vi "2022NewInstrumentationU6Revision.vi"() -> ()   [LabVIEW 2021]
uses:
  <vilib>/Analysis/baseanly.llb/Mean (DBL).vi
  <vilib>/Analysis/NI_AALBase.lvlib
panel:
  out "Combustion Chamber Pressure":dbl(knob) scale=0.0..10.0
  out "Pre-Injector Pressure":dbl(graph)
  out "Post-Combustion Chamber Temperature":dbl(knob) scale=0.0..10.0
  out "Pre-Combustion Chamber Temperature":dbl(knob) scale=0.0..100.0
  out "Injector Temperature":dbl(knob) scale=0.0..10.0
  out "Run Tank: Temperature":dbl(slide) scale=0.0..100.0
  out "Run Tank: Pressure":dbl(knob) scale=0.0..10.0
  out "N20 Post-Tank: Pressure":dbl(knob) scale=0.0..10.0
  out "N2 Post-tank: Pressure":dbl(knob) scale=0.0..10.0
  in  "file name":string
  in  "file path":path
  in  "Iterations/Second":i32=1
  in  "Binary":bool
  in  "StreamSettlingFactor":i32
  in  "Resolution Index":u8
  in  "Range Constants":u8[](array[ring])=[0, 0, 0, 0] items=["LJ_rgBIP10V", "LJ_rgBIP1V", "LJ_rgBIPP1V", "LJ_rgBIPP01V"]
  out "Stream Parameters":T1 {"Device Backlog [%]" format="%.2f"}
  in  "PC buffer size (seconds)":dbl=10.0 format="%.2f"
  in  "Scan List (-)":u8[](array[numeric])=[199, 199, 199, 199]
  in  "Scan List (+)":u8[](array[numeric])=[0, 1, 2, 3]
  out "# of iterations":i32
  in  "Scan Rate (Hz)":dbl=1000.0 format="%.3f"
  in  "stop":bool
  out "Error Message":string
  # "This example streams from the first found USB U6."
  # "The + scan list is the positive\nchannels.  For each element in\nthe + list, there must also be\nan element in the - list, which is\nthe negative channels.  For\nsingle-ended channels, put in\n199 for the negative channel.\n\nTo remove an element, right-click\non it, select Data Operations =>\nRemove Element.\n\nTo empty an array, right-click\nnear the edge, select Data\nOperations => Empty Array.\n\nOther useful operations:  From the\nOperate menu are \"Make Current\nValues Default\" and \"Reinitialize\nTo Default\"."
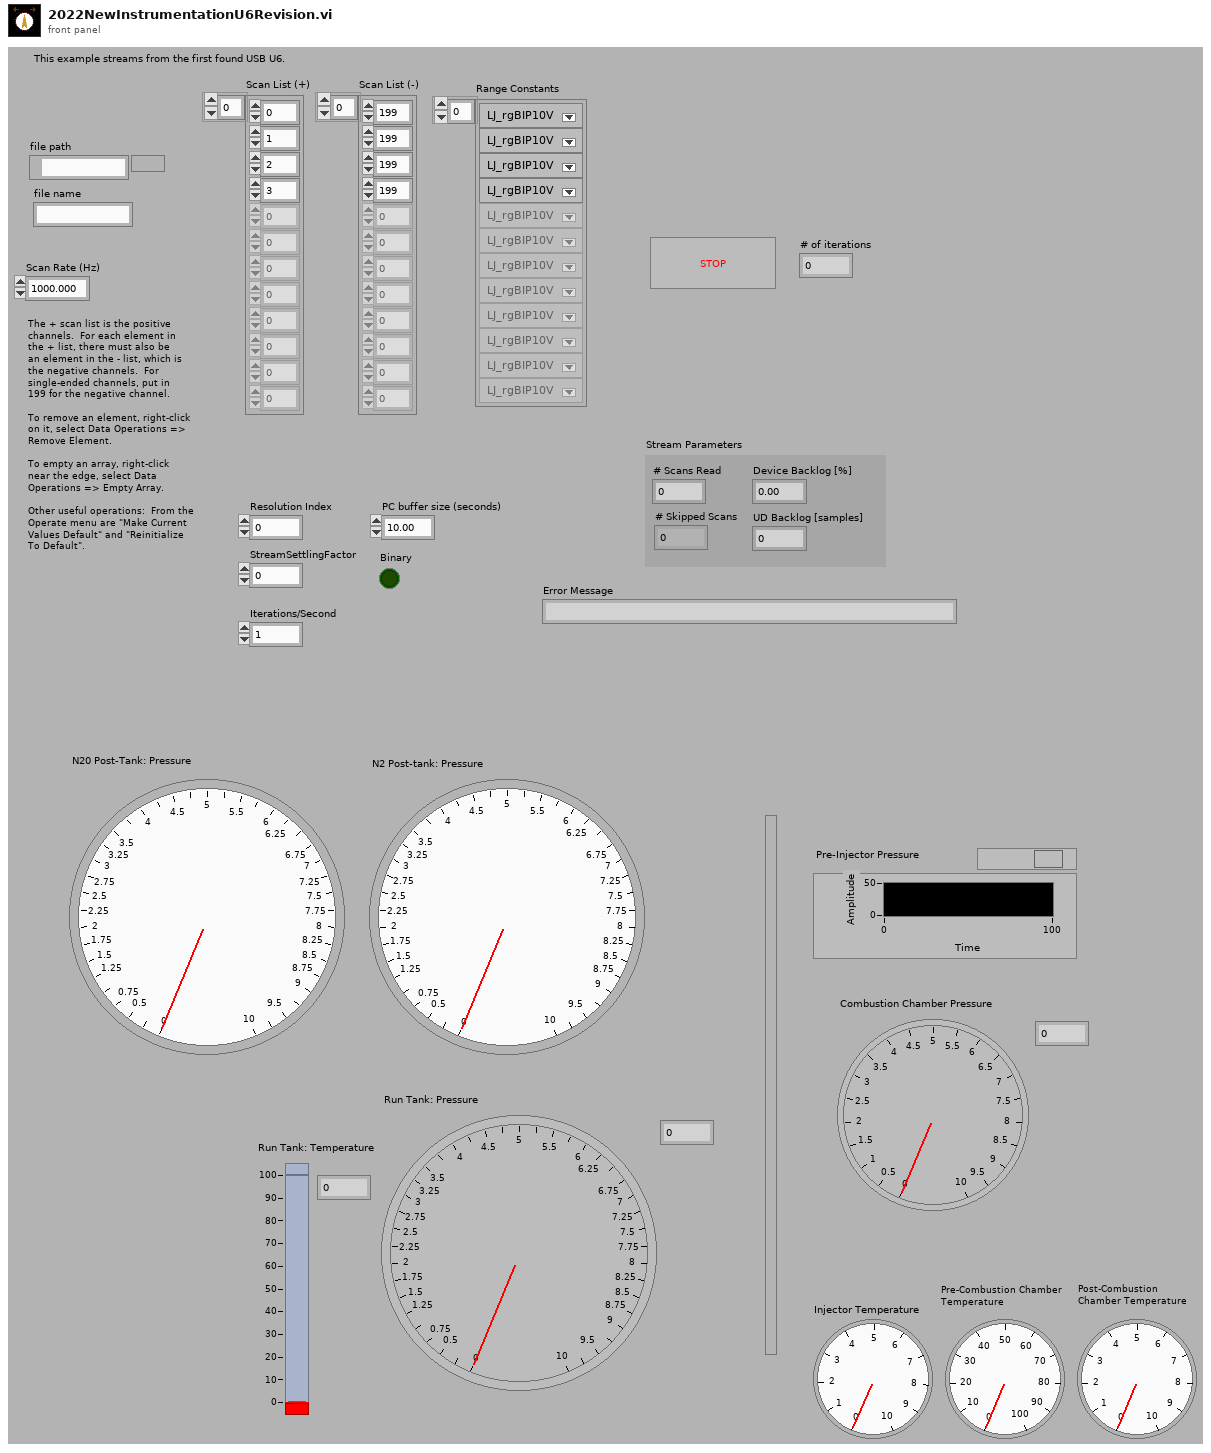
[diagram p1: front panel]
types:
  T1 = cluster{"# Scans Read":i32, "# Skipped Scans":i32, "Device Backlog [%]":dbl, "UD Backlog [samples]":i32}
  T2 = enum16{"open", "open or create", "create or replace", "create", "open (read-only)"}
  T3 = cluster{"PC buffer size (seconds)":dbl, "Resolution Index":u8, "StreamSettlingFactor":i32, "Binary":bool}
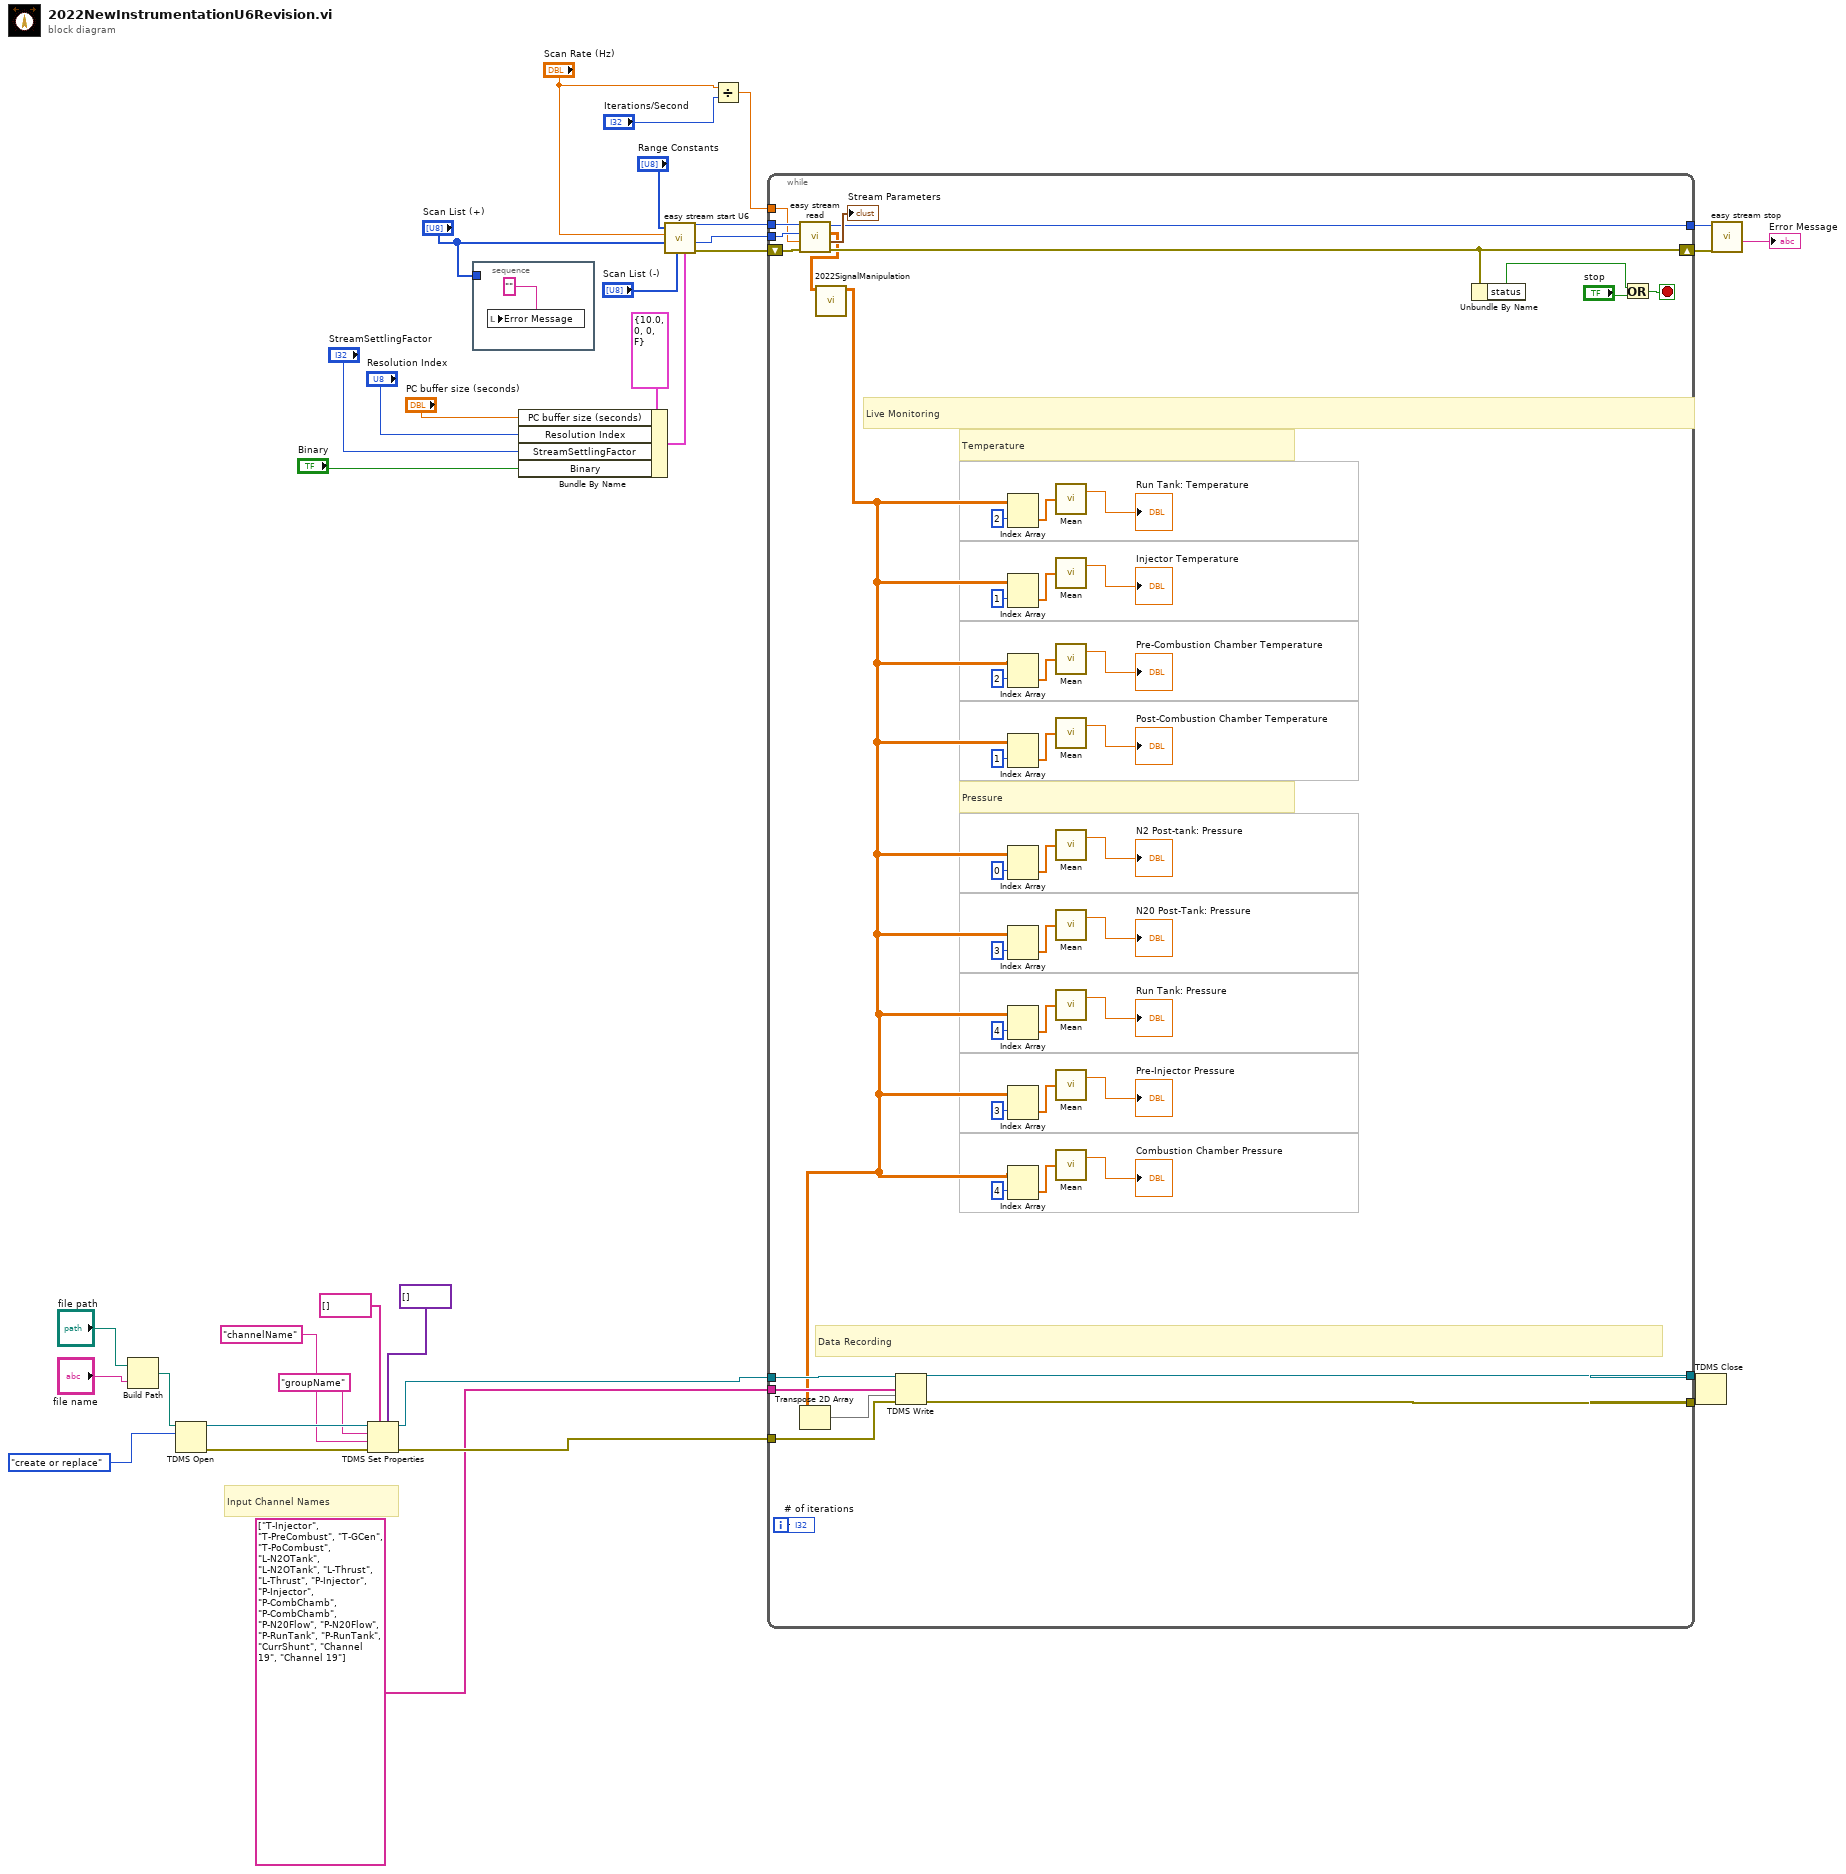
[diagram p0: block diagram]
diagram:
  # "Input Channel Names"
  n1 = Build Path(base path="file path", name or relative path="file name") -> (appended path=w11:path)
  n2 = TDMS Open(10:T2."create or replace" ("operation (0:open)"), 11:w11) -> (0:w16:errorcluster, 3:w15:refnum<k34>)  [unwired: 5 in]
  n3 = TDMS Set Properties(5:variant[] [] ("property values"), 7:string[] [] ("property names"), 8:w16, 9:"channelName" ("channel name"), 10:"groupName" ("group name"), 11:w15) -> (0:w6:errorcluster, 3:w5:refnum<k34>)  [unwired: 2 out]
  n4 = stacked-sequence {
    tunnel: "Scan List (+)" -> [_]
    frame #0 {
      n5 = local write "Error Message"("" ("Error Message")) -> ()
    }
  }
  n6 = Bundle By Name(cluster=T3 {"PC buffer size (seconds)"=10.0, "Resolution Index"=0, "StreamSettlingFactor"=0, "Binary"=FALSE} ("Advanced"), "PC buffer size (seconds)"="PC buffer size (seconds)", "Resolution Index"="Resolution Index", "StreamSettlingFactor"="StreamSettlingFactor", "Binary"="Binary") -> (w24:T3)
  n7 = call "easy stream start U6.vi"("Advanced"=w24, "Scan List (-)"="Scan List (-)", "Scan List (+)"="Scan List (+)", "Scan Rate (Hz)"="Scan Rate (Hz)", "Range Constants"="Range Constants") -> ("error out"=w33:errorcluster, "# Channels"=w32:i32, "Handle Out"=w31:i32)  [unwired: 3 in, 1 out]
  n8 = Divide(x="Scan Rate (Hz)", y="Iterations/Second") -> (x/y=w17:dbl)
  n9 = while {
    tunnel: w31 -> [w74]
    tunnel: w32 -> [w75]
    shift-left: w33 -> [w76]
    shift-right: [w56] -> w30
    tunnel: w17 -> [w72]
    tunnel: w6 -> [w71]
    tunnel: w5 -> [w70]
    tunnel: string[] ["T-Injector", "T-PreCombust", "T-GCen", "T-PoCombust", "L-N2OTank", "L-N2OTank", "L-Thrust", "L-Thrust", "P-Injector", "P-Injector", "P-CombChamb", "P-CombChamb", "P-N20Flow", "P-N20Flow", "P-RunTank", "P-RunTank", "CurrShunt", "Channel 19", "Channel 19"] -> [w69]
    tunnel: [w68] -> w3
    tunnel: [w67] -> w2
    tunnel: [w55] -> w1
    i -> [w77]
    stop <- w78 stop-if-true
    # "Data Recording"
    # "Temperature"
    # "Live Monitoring"
    # "Pressure"
    n10 = call "easy stream read.vi"("error in"=w76, "Scans To Read"=w72, "# Channels In Stream"=w75, "Handle In"=w74) -> ("error out"=w56:errorcluster, "Stream Parameters"=→"Stream Parameters":T1, "Data"=w54:dbl[][], "Handle Out"=w55:i32)  [unwired: 4 in]
    n11 = call "2022SignalManipulation.vi"("Data"=w54) -> ("Array"=w36:dbl[][])  [unwired: 10 in]
    n12 = Transpose 2D Array(2D array=w36) -> (transposed array=w66:dbl[][])
    n13 = TDMS Write(0:w70, 7:w69, 9:w66, 11:w71) -> (4:w67:refnum<k34>, 15:w68:errorcluster)  [unwired: 2 in, 2 out]
    n14 = Index Array(array=w36, index (col)=2) -> (element=w53:dbl[])  [unwired: 1 in]
    n15 = Index Array(array=w36, index (col)=1) -> (element=w52:dbl[])  [unwired: 1 in]
    n16 = Index Array(array=w36, index (col)=2) -> (element=w43:dbl[])  [unwired: 1 in]
    n17 = Index Array(array=w36, index (col)=1) -> (element=w42:dbl[])  [unwired: 1 in]
    n18 = Index Array(array=w36, index (col)=0) -> (element=w51:dbl[])  [unwired: 1 in]
    n19 = Index Array(array=w36, index (col)=3) -> (element=w50:dbl[])  [unwired: 1 in]
    n20 = Index Array(array=w36, index (col)=4) -> (element=w49:dbl[])  [unwired: 1 in]
    n21 = Index Array(array=w36, index (col)=3) -> (element=w37:dbl[])  [unwired: 1 in]
    n22 = Index Array(array=w36, index (col)=4) -> (element=w35:dbl[])  [unwired: 1 in]
    n23 = call-poly <vilib>:"Mean.vi"("X"=w53) -> ("mean"=→"Run Tank: Temperature":dbl)  [unwired: 1 out]
    n24 = call-poly <vilib>:"Mean.vi"("X"=w52) -> ("mean"=→"Injector Temperature":dbl)  [unwired: 1 out]
    n25 = call-poly <vilib>:"Mean.vi"("X"=w43) -> ("mean"=→"Pre-Combustion Chamber Temperature":dbl)  [unwired: 1 out]
    n26 = call-poly <vilib>:"Mean.vi"("X"=w42) -> ("mean"=→"Post-Combustion Chamber Temperature":dbl)  [unwired: 1 out]
    n27 = call-poly <vilib>:"Mean.vi"("X"=w51) -> ("mean"=→"N2 Post-tank: Pressure":dbl)  [unwired: 1 out]
    n28 = call-poly <vilib>:"Mean.vi"("X"=w50) -> ("mean"=→"N20 Post-Tank: Pressure":dbl)  [unwired: 1 out]
    n29 = call-poly <vilib>:"Mean.vi"("X"=w49) -> ("mean"=→"Run Tank: Pressure":dbl)  [unwired: 1 out]
    n30 = call-poly <vilib>:"Mean.vi"("X"=w37) -> ("mean"=→"Pre-Injector Pressure":dbl)  [unwired: 1 out]
    n31 = call-poly <vilib>:"Mean.vi"("X"=w35) -> ("mean"=→"Combustion Chamber Pressure":dbl)  [unwired: 1 out]
    n32 = Unbundle By Name(w56) -> ("status"=w79:bool)
    n33 = Or(x=w79, y="stop") -> (x .or. y?=w78:bool)
    "# of iterations" <- w77
  }
  n34 = TDMS Close(8:w3, 11:w2) -> ()  [unwired: 2 out]
  n35 = call "easy stream stop.vi"("error in"=w30, "Handle In"=w1) -> ("Error Message"=→"Error Message":string)  [unwired: 7 in, 2 out]
